vi "SetLeftSize.vi"(8 "error in (no error)":errorcluster, 10 "Left Pane Size":i32, 11 "PentaPanesGUI in":refnum<class "PentaPanes.lvclass">) -> (0 "error out":errorcluster, 3 "PentaPanesGUI out":refnum<class "PentaPanes.lvclass">)   [LabVIEW 2022 SP3, in "PentaPanesLibrary.lvlib" / "PentaPanes.lvclass"]
doc: "This VI sets the width of the Left pane.\n\nLeft Pane Size - The width of the pane to be set."
uses:
  PentaPanes.lvclass
  PentaPanes.lvclass/PentaPanes.ctl
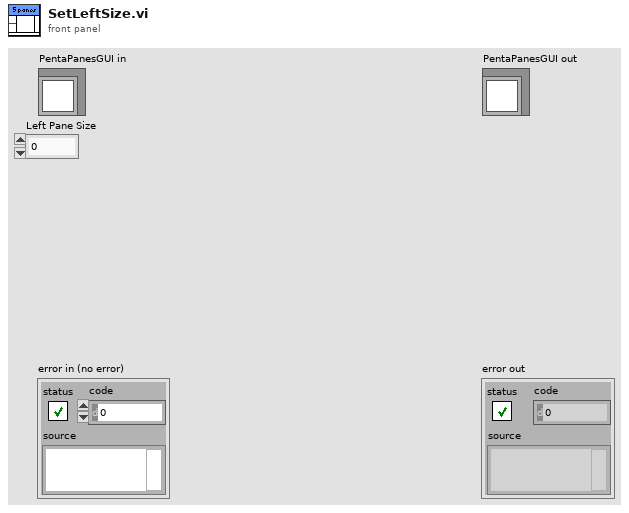
[diagram p1: front panel]
types:
  T1 = typedef "PentaPanesLibrary.lvlib/PentaPanes.lvclass/SplittersCluster.ctl" = cluster{"Top Splitter":refnum<vi>, "Left Splitter":refnum<vi>, "Right Splitter":refnum<vi>, "Bottom Splitter":refnum<vi>}
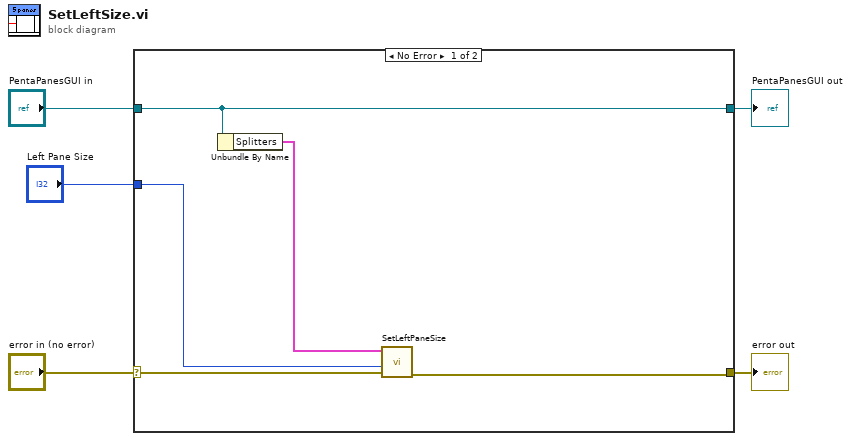
[diagram p0: block diagram]
diagram:
  n1 = case shown="No Error" "error in (no error)" {
    selector: "error in (no error)" -> [w7 w12]
    tunnel: [w6 w12] -> w4
    tunnel: [w10 w11] -> w2
    tunnel: "PentaPanesGUI in" -> [w10 w11]
    tunnel: "Left Pane Size" -> [w8 _]
    frame No Error {
      n2 = Unbundle By Name(w10) -> ("Splitters"=w9:T1)
      n3 = call "SetLeftPaneSize.vi"("error in (no error)"=w7, "Left Pane Size"=w8, "Splitters"=w9) -> ("error out"=w6:errorcluster)  [unwired: 8 in]
    }
    frame Error {
    }
  }
  "error out" <- w4
  "PentaPanesGUI out" <- w2
